vi "short_cmd_write.vi"(5 "COM":bool, 7 "VISA name":refnum<visa-resource-name>, 8 "data":u8[](array[numeric]), 9 "dwLen":u16, 10 "dwAddr":u16, 11 "cmd_short_header_t":T1) -> (3 "return":i32)   [LabVIEW 2016]
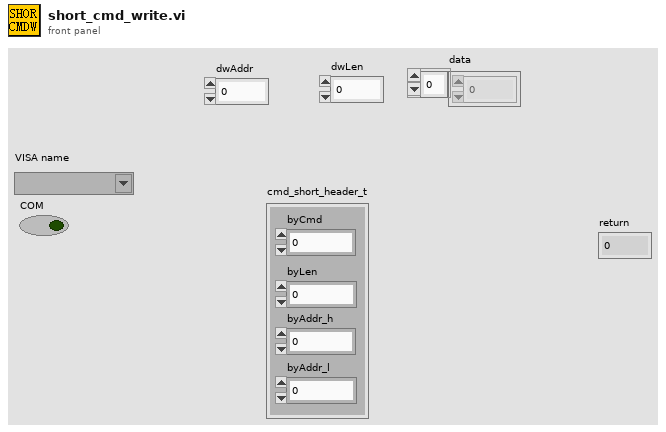
[diagram p1: front panel]
types:
  T1 = cluster{"byCmd":u8, "byLen":u8, "byAddr_h":u8, "byAddr_l":u8}
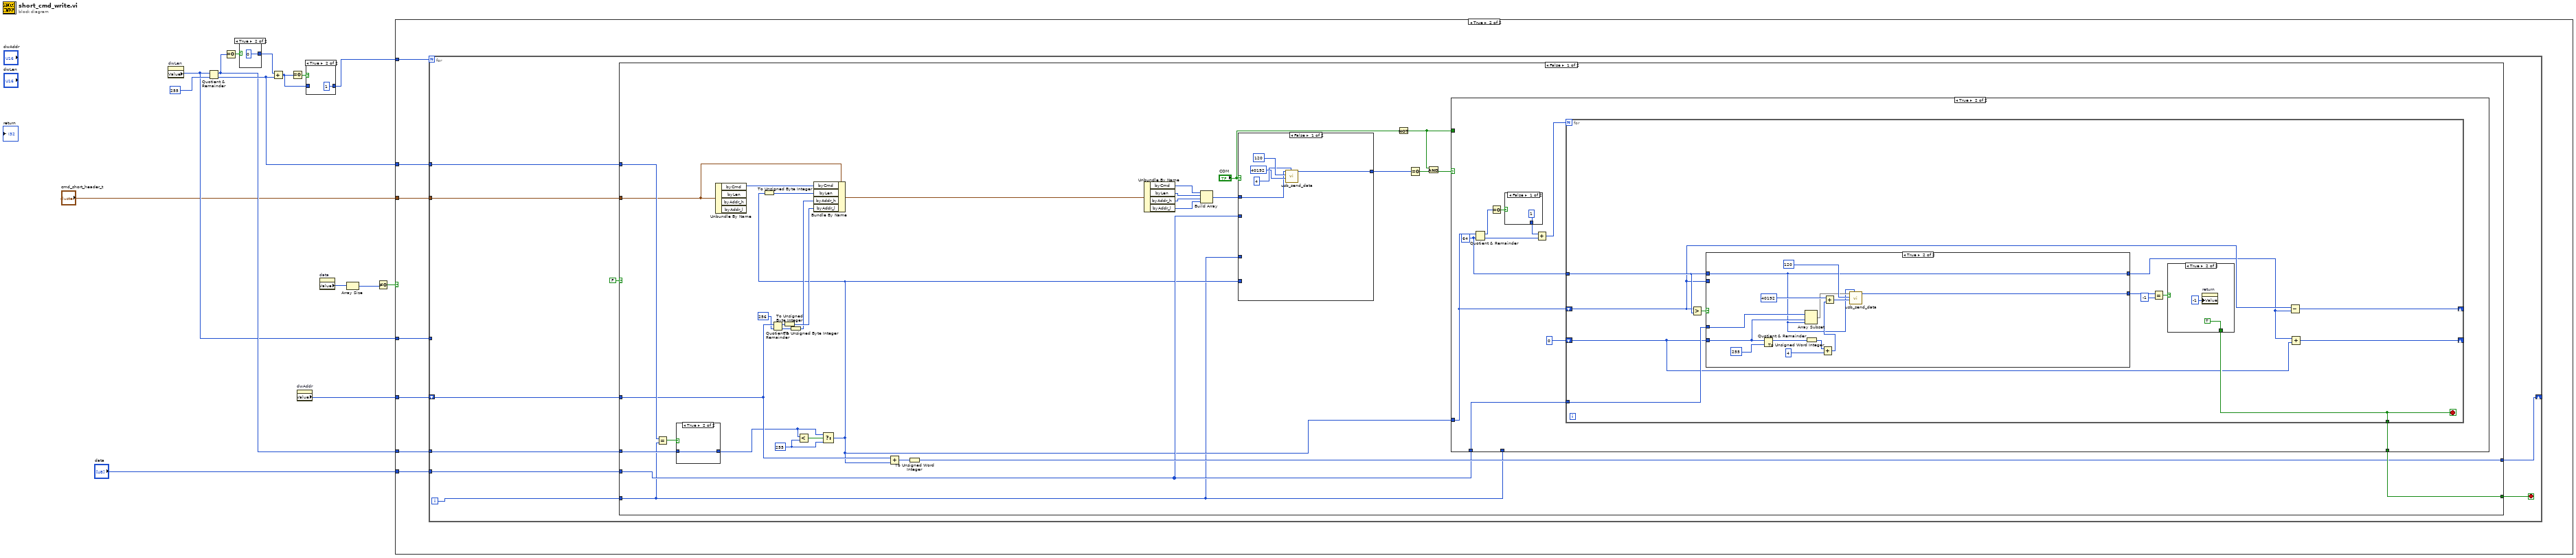
[diagram p0: block diagram]
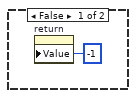
[diagram p2: hidden frame]
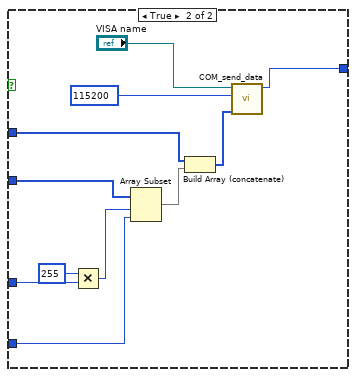
[diagram p3: hidden frame]
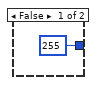
[diagram p4: hidden frame]
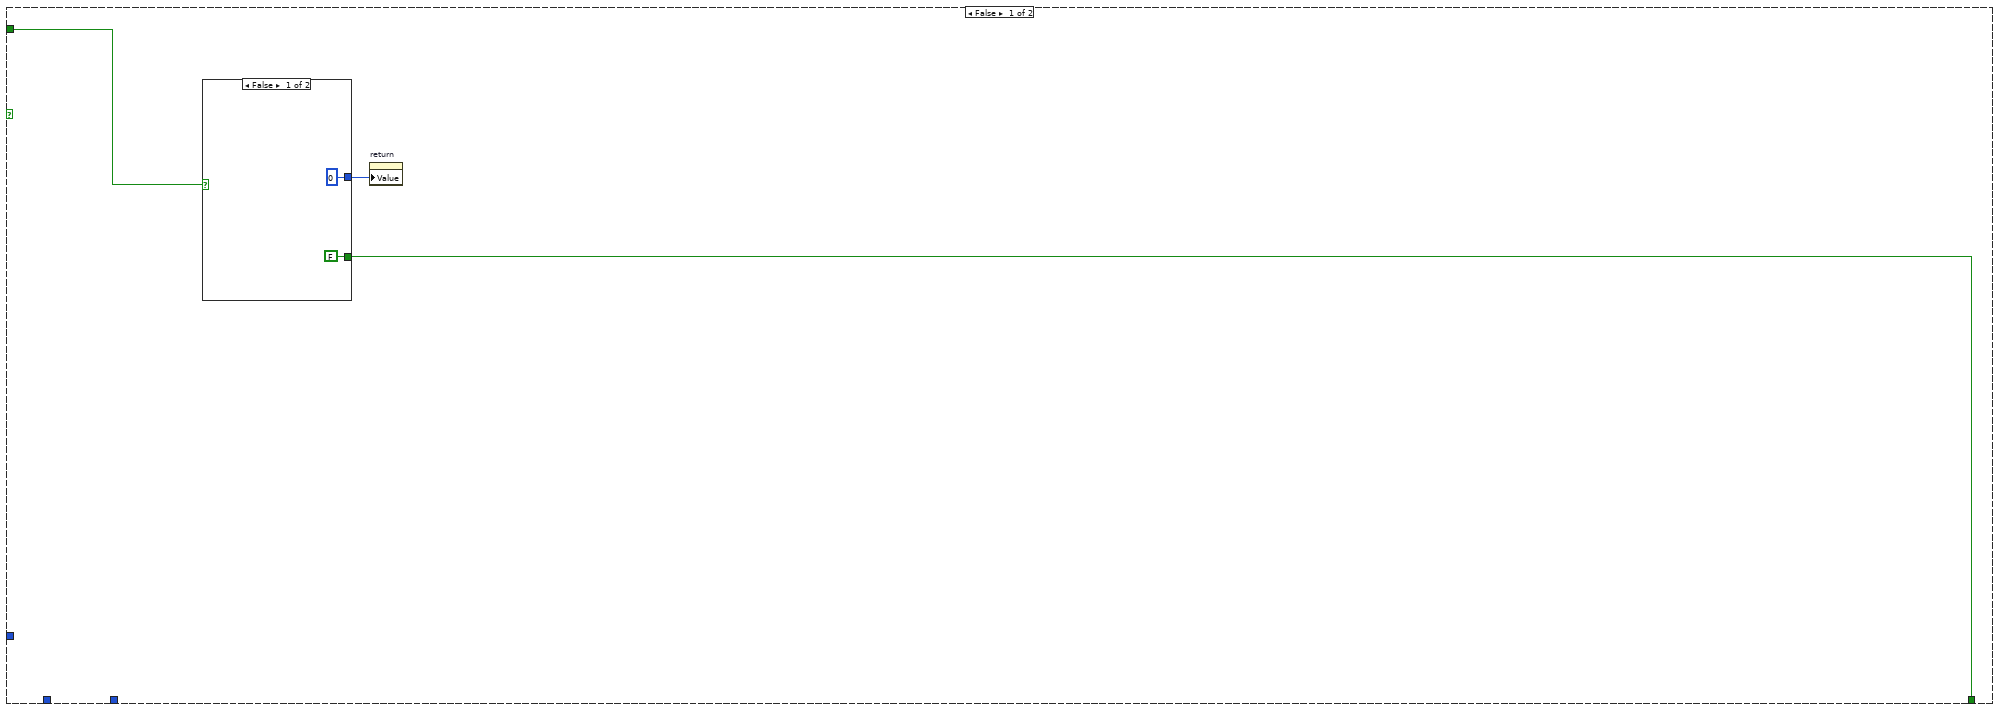
[diagram p5: hidden frame]
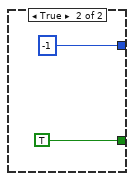
[diagram p6: hidden frame]
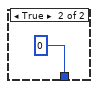
[diagram p7: hidden frame]
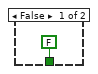
[diagram p8: hidden frame]
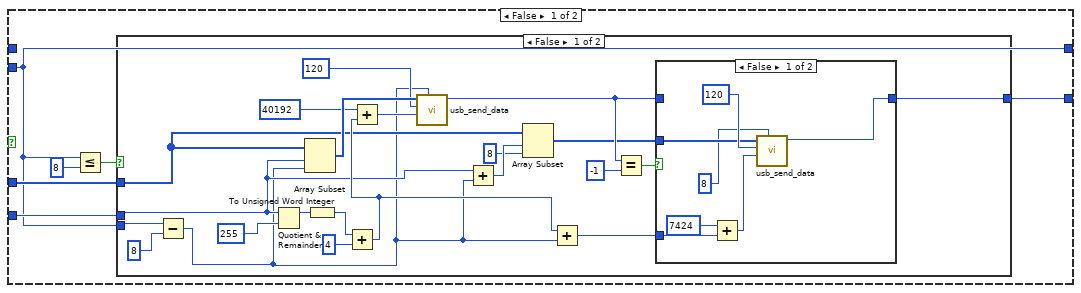
[diagram p9: hidden frame]
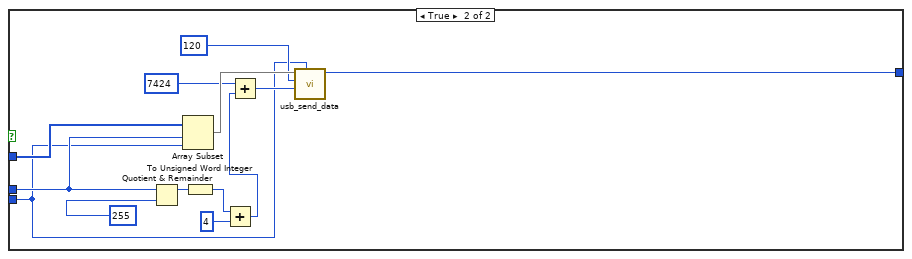
[diagram p11: hidden frame]
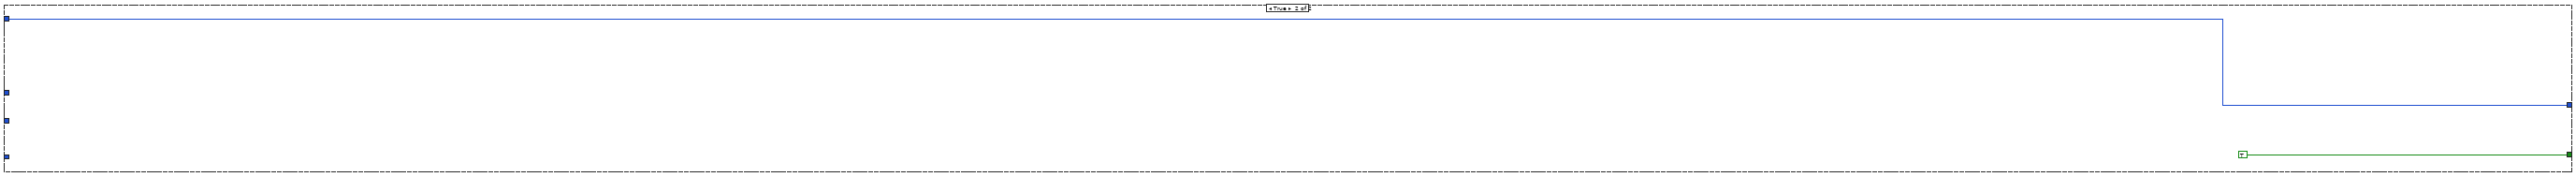
[diagram p12: hidden frame]
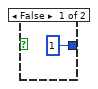
[diagram p14: hidden frame]
diagram:
  n1 = property on="dwLen" class="DigNum (strict)"() -> ("Value"=w8:u16)  [unwired: 2 in, 2 out]
  n2 = Quotient & Remainder(x=w8, y=u16 255) -> (x-y*floor(x/y)=w11:u16, floor(x/y)=w12:u16)
  n3 = Equal To 0?(x=w11) -> (x = 0?=w14:bool)
  n4 = case shown="True" w14 {
    tunnel: [u16 1 u16 0] -> w13
    frame False {
    }
    frame True {
    }
  }
  n5 = Add(x=w13, y=w12) -> (x+y=w5:u16)
  n6 = Equal To 0?(x=w5) -> (x = 0?=w6:bool)
  n7 = property on="dwAddr" class="DigNum (strict)"() -> ("Value"=w9:u16)  [unwired: 2 in, 2 out]
  n8 = case shown="True" w6 {
    tunnel: w5 -> [w18 _]
    tunnel: [w18 u16 1] -> w4
    frame False {
    }
    frame True {
    }
  }
  n9 = property on="data" class="Arr (strict)"() -> ("Value"=w7:u8[])  [unwired: 2 in, 2 out]
  n10 = Array Size(array=w7) -> (size(s)=w2:i32)
  n11 = Not Equal To 0?(x=w2) -> (x != 0?=w3:bool)
  n12 = case shown="True" w3 {
    tunnel: w12 -> [_ w27]
    tunnel: w11 -> [_ w26]
    tunnel: "data" -> [_ w25]
    tunnel: w9 -> [_ w24]
    tunnel: w8 -> [_ w23]
    tunnel: w4 -> [_ w22]
    tunnel: "cmd_short_header_t" -> [_ w21]
    frame False {
      n13 = property on="return" class="DigNum (strict)"("Value"=-1 ("return")) -> ()  [unwired: 2 in, 2 out]
    }
    frame True {
      n14 = for {
        N: w22 -> [_]
        tunnel: w27 -> [w35]
        tunnel: w26 -> [w34]
        shift-right: [w32] -> _
        shift-left: w24 -> [w33]
        tunnel: w23 -> [_]
        tunnel: w25 -> [w31]
        tunnel: w21 -> [w28]
        i -> [w30]
        stop <- w36 stop-if-true
        n15 = case shown="False" FALSE {
          tunnel: [w65 TRUE] -> w36
          tunnel: w35 -> [w63 _]
          tunnel: w34 -> [w62 _]
          tunnel: w33 -> [w59 w183]
          tunnel: [w44 w183] -> w32
          tunnel: w31 -> [w42 _]
          tunnel: w30 -> [w40 _]
          tunnel: w28 -> [w57 _]
          frame False {
            w67 = u16 255 ("f")
            n16 = Equal?(x=w63, y=w40) -> (x = y?=w64:bool)
            n17 = case shown="True" w64 {
              tunnel: w62 -> [_ w86]
              tunnel: [u16 255 w86] -> w43
              frame False {
              }
              frame True {
              }
            }
            n18 = Unbundle By Name(w57) -> ("byCmd"=w51:u8)  [unwired: 3 out]
            n19 = Quotient & Remainder(x=w59, y=u16 256) -> (x-y*floor(x/y)=w56:u16, floor(x/y)=w54:u16)
            n20 = To Unsigned Byte Integer(number=w56) -> (unsigned 8bit integer=w55:u8)
            n21 = To Unsigned Byte Integer(number=w54) -> (unsigned 8bit integer=w53:u8)
            n22 = Less?(x=w43, y=w67) -> (x < y?=w68:bool)
            n23 = Select(t=w43, s=w68, f=w67) -> (s? t:f=w41:u16)
            n24 = To Unsigned Byte Integer(number=w41) -> (unsigned 8bit integer=w52:u8)
            n25 = Bundle By Name(cluster=w57, "byCmd"=w51, "byLen"=w52, "byAddr_h"=w53, "byAddr_l"=w55) -> (w50:T1)
            n26 = Add(x=w59, y=w41) -> (x+y=w61:u16)
            n27 = To Unsigned Word Integer(number=w61) -> (unsigned 16bit integer=w44:u16)
            n28 = Unbundle By Name(w50) -> ("byCmd"=w49:u8, "byLen"=w48:u8, "byAddr_h"=w47:u8, "byAddr_l"=w46:u8)
            n29 = Build Array(w49, w48, w47, w46) -> (w45:u8[])
            n30 = case shown="False" "COM" {
              tunnel: [w71 w76] -> w60
              tunnel: w45 -> [w70 w78]
              tunnel: w42 -> [_ w79]
              tunnel: w41 -> [_ w81]
              tunnel: w40 -> [_ w80]
              frame False {
                n31 = call "usb_send_data.vi"("byVdCmdHeaderLen"=u16 4, "I2C_VD_BUFFER_RW"=u16 40192, "I2C_SLAVE_ID"=u8 120, "data"=w70) -> ("return"=w71:i32)  [unwired: 6 in, 1 out]
              }
              frame True {
                n32 = Multiply(x=255, y=w80) -> (x*y=w84:i32)
                n33 = Array Subset(array=w79, index=w84, length=w81) -> (w83:u8[])
                n34 = Build Array (concatenate)(w78, w83) -> (w77:u8[])
                n35 = call "COM_send_data.vi"("data"=w77, "baud rate (9600)"=u32 115200, "VISA name"="VISA name") -> ("return"=w76:i32)  [unwired: 8 in]
              }
            }
            n36 = Not(x="COM") -> (.not. x?=w37:bool)
            n37 = Equal To 0?(x=w60) -> (x = 0?=w66:bool)
            n38 = And(x=w37, y=w66) -> (x .and. y?=w39:bool)
            n39 = case shown="True" w39 {
              tunnel: [w88 w95] -> w65
              tunnel: w41 -> [_ w98]
              tunnel: w42 -> [_ w94]
              tunnel: w40 -> [_ _]
              tunnel: w37 -> [w87 _]
              frame False {
                n40 = case shown="False" w87 {
                  tunnel: [0 ("return") -1 ("return")] -> w89
                  tunnel: [FALSE TRUE] -> w88
                  frame False {
                  }
                  frame True {
                  }
                }
                n41 = property on="return" class="DigNum (strict)"("Value"=w89) -> ()  [unwired: 2 in, 2 out]
              }
              frame True {
                w97 = u16 64 ("y")
                n42 = Quotient & Remainder(x=w98, y=w97) -> (x-y*floor(x/y)=w102:u16, floor(x/y)=w100:u16)
                n43 = Equal To 0?(x=w102) -> (x = 0?=w103:bool)
                n44 = case shown="False" w103 {
                  tunnel: [u32 1 ("x-y*floor(x/y)") u32 0 ("x-y*floor(x/y)")] -> w101
                  frame False {
                  }
                  frame True {
                  }
                }
                n45 = Add(x=w101, y=w100) -> (x+y=w99:u32)
                n46 = for {
                  N: w99 -> [_]
                  shift-right: [w106] -> _
                  shift-left: w98 -> [w110]
                  tunnel: w97 -> [w116]
                  shift-right: [w107] -> _
                  shift-left: u32 0 -> [w108]
                  tunnel: w94 -> [w115]
                  tunnel: [w111] -> w95
                  stop <- w111 stop-if-true
                  n47 = Greater?(x=w110, y=w116) -> (0:w117:bool)
                  n48 = case shown="True" w117 {
                    tunnel: w116 -> [_ w170]
                    tunnel: w110 -> [w122 _]
                    tunnel: [w122 w170] -> w109
                    tunnel: w108 -> [w125 w173]
                    tunnel: w115 -> [w124 w175]
                    tunnel: [w126 w171] -> w113
                    frame False {
                      n49 = Less Or Equal?(x=w122, y=u32 8) -> (x <= y?=w123:bool)
                      n50 = case shown="False" w123 {
                        tunnel: [w137 w161] -> w126
                        tunnel: w125 -> [w133 w160]
                        tunnel: w124 -> [w130 w159]
                        tunnel: w122 -> [w141 w157]
                        frame False {
                          n51 = Subtract(x=w141, y=u32 8) -> (x-y=w127:u32)
                          n52 = Quotient & Remainder(x=w133, y=u32 255) -> (x-y*floor(x/y)=w147:u32)  [unwired: 1 out]
                          n53 = Array Subset(array=w130, index=w133, length=w127) -> (w145:u8[])
                          n54 = To Unsigned Word Integer(number=w147) -> (unsigned 16bit integer=w146:u16)
                          n55 = Add(x=w146, y=u16 4) -> (x+y=w135:u16)
                          n56 = Add(x=u16 40192 ("I2C_VD_BUFFER_RW"), y=w135) -> (x+y=w148:u16)
                          n57 = call "usb_send_data.vi"("byVdCmdHeaderLen"=w127, "I2C_VD_BUFFER_RW"=w148, "I2C_SLAVE_ID"=u8 120, "data"=w145) -> ("return"=w136:i32)  [unwired: 6 in, 1 out]
                          n58 = Add(x=w133, y=w127) -> (x+y=w132:u32)
                          n59 = Array Subset(array=w130, index=w132, length=8) -> (w129:u8[])
                          n60 = Add(x=w135, y=w127) -> (x+y=w134:u32)
                          n61 = Equal?(x=w136, y=-1) -> (x = y?=w139:bool)
                          n62 = case shown="False" w139 {
                            tunnel: [w155 w156] -> w137
                            tunnel: w136 -> [_ w156]
                            tunnel: w134 -> [w154 _]
                            tunnel: w129 -> [w150 _]
                            frame False {
                              n63 = Add(x=u32 7424, y=w154) -> (x+y=w153:u32)
                              n64 = call "usb_send_data.vi"("byVdCmdHeaderLen"=u16 8, "I2C_VD_BUFFER_RW"=w153, "I2C_SLAVE_ID"=u8 120, "data"=w150) -> ("return"=w155:i32)  [unwired: 6 in, 1 out]
                            }
                            frame True {
                            }
                          }
                        }
                        frame True {
                          n65 = Quotient & Remainder(x=w160, y=u32 255) -> (x-y*floor(x/y)=w168:u32)  [unwired: 1 out]
                          n66 = Array Subset(array=w159, index=w160, length=w157) -> (w165:u8[])
                          n67 = To Unsigned Word Integer(number=w168) -> (unsigned 16bit integer=w167:u16)
                          n68 = Add(x=w167, y=u16 4) -> (x+y=w166:u16)
                          n69 = Add(x=u16 7424 ("I2C_VD_BUFFER_RW"), y=w166) -> (x+y=w169:u16)
                          n70 = call "usb_send_data.vi"("byVdCmdHeaderLen"=w157, "I2C_VD_BUFFER_RW"=w169, "I2C_SLAVE_ID"=u8 120, "data"=w165) -> ("return"=w161:i32)  [unwired: 6 in, 1 out]
                        }
                      }
                    }
                    frame True {
                      n71 = Quotient & Remainder(x=w173, y=u32 255) -> (x-y*floor(x/y)=w179:u32)  [unwired: 1 out]
                      n72 = Array Subset(array=w175, index=w173, length=w170) -> (w172:u8[])
                      n73 = To Unsigned Word Integer(number=w179) -> (unsigned 16bit integer=w178:u16)
                      n74 = Add(x=w178, y=u16 4) -> (x+y=w176:u16)
                      n75 = Add(x=u16 40192 ("I2C_VD_BUFFER_RW"), y=w176) -> (x+y=w181:u16)
                      n76 = call "usb_send_data.vi"("byVdCmdHeaderLen"=w170, "I2C_VD_BUFFER_RW"=w181, "I2C_SLAVE_ID"=u8 120, "data"=w172) -> ("return"=w171:i32)  [unwired: 6 in, 1 out]
                    }
                  }
                  n77 = Equal?(x=w113, y=-1) -> (x = y?=w114:bool)
                  n78 = case shown="True" w114 {
                    tunnel: [FALSE TRUE] -> w111
                    frame False {
                    }
                    frame True {
                      n79 = property on="return" class="DigNum (strict)"("Value"=-1 ("return")) -> ()  [unwired: 2 in, 2 out]
                    }
                  }
                  n80 = Subtract(x=w110, y=w109) -> (x-y=w106:u16)
                  n81 = Add(x=w109, y=w108) -> (x+y=w107:u32)
                }
              }
            }
          }
          frame True {
          }
        }
      }
    }
  }
